vi "New SequenceFile.vi"(8 "error in (no error)":errorcluster) -> (0 "error out":errorcluster, 3 "SequenceFile out":refnum<class "SequenceFile.lvclass">)   [LabVIEW 2020, in "TSnax.lvlib" / "SequenceFile.lvclass"]
uses:
  SequenceFile.lvclass
  SequenceFile.lvclass/SequenceFile.ctl
  Engine/Engine.lvclass
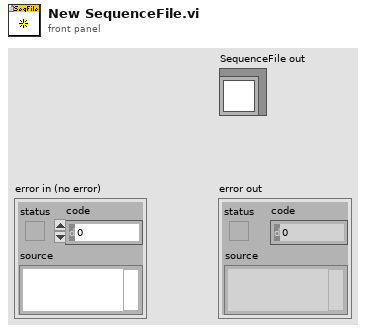
[diagram p1: front panel]
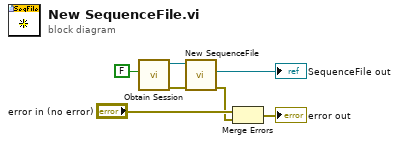
[diagram p0: block diagram]
diagram:
  n1 = call "Obtain Session.vi"("Create if needed? (T)"=FALSE) -> ("error out"=w5:errorcluster, "Engine out"=w4:refnum<class "Engine.lvclass">)  [unwired: 9 in]
  n2 = call "New SequenceFile.vi"("error in (no error)"=w5, "Engine in"=w4) -> ("error out"=w1:errorcluster, "New SequenceFile"=→"SequenceFile out":refnum<class "SequenceFile.lvclass">)  [unwired: 7 in, 1 out]
  n3 = Merge Errors("error in (no error)", w1) -> (→"error out":errorcluster)
